vi "estop_fgv.vi"(8 "error in (no error)":errorcluster, 9 "Boolean":bool, 11 "Enum":enum16{"set", "get"}(ring)) -> (0 "error out":errorcluster, 1 "indicator":bool)   [LabVIEW 2019]
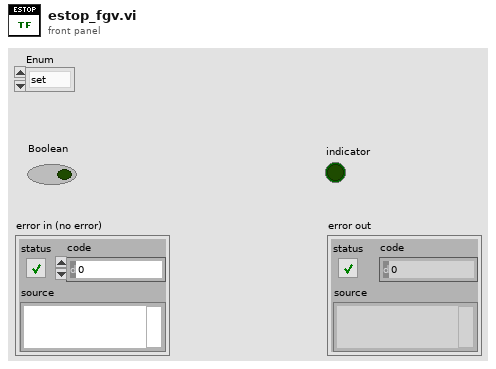
[diagram p1: front panel]
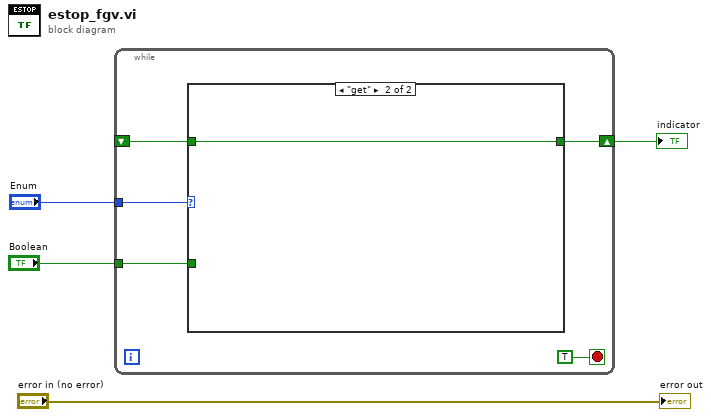
[diagram p0: block diagram]
diagram:
  n1 = while {
    tunnel: "Enum" -> [w9]
    tunnel: "Boolean" -> [w7]
    shift-right: [w8] -> w2
    shift-left: _ -> [w6]
    stop <- TRUE stop-if-true
    n2 = case shown="\"get\"" w9 {
      tunnel: [w10 w11] -> w8
      tunnel: w7 -> [w10 _]
      tunnel: w6 -> [_ w11]
      frame "set", Default {
      }
      frame "get" {
      }
    }
  }
  "indicator" <- w2
  "error out" <- "error in (no error)"
